vi "ctrlMain.vi"() -> ()   [LabVIEW 2012]
panel:
  out "Label":string
  in  "InitDevices":bool
  out "数值":i32
  out "remote address":string caption="远程地址"
  out "remote port":u16 caption="远程端口"
  out "data out":string
  in  "StopTCP":bool
  in  "StopLoop":bool
  out "status changed":string
  out "REDY_THL5":bool caption="THL5"
  out "REDY_THL3":bool caption="THL3"
  out "REDY_THL6":bool caption="THL6"
  out "REDY_THL4":bool caption="THL4"
  out "REDY_THL2":bool caption="THL2"
  out "REDY_THL1":bool caption="THL1"
  out "REDY_PIZ":bool caption="PIZ"
  out "REDY_NPR":bool caption="NPR"
  out "REDY_NPM":bool caption="NPM"
  in  "选项卡控件 2":T1(tab)
  out "sz":bool
  out "sy":bool
  out "sx":bool
  in  "pz":dbl
  in  "py":dbl
  in  "px":dbl
  out "pxd":dbl
  in  "Sample_speed":dbl(slide) scale=0.01..10.0
  in  "x-":bool
  in  "x+":bool
  in  "y+":bool
  in  "y-":bool
  in  "z-":bool
  in  "z+":bool
  out "pyd":dbl
  out "pzd":dbl
  out "sM2y":bool
  out "sM2x":bool
  out "sM1y":bool
  out "sM1x":bool
  in  "M2xp":dbl
  in  "M1yp":dbl
  in  "M1xp":dbl
  out "M1xpd":dbl
  in  "M_speed":i16(slide) scale=10.0..2000.0
  in  "M1x-":bool
  in  "M1x+":bool
  in  "M1y+":bool
  in  "M1y-":bool
  in  "M2x-":bool
  in  "M2x+":bool
  out "M1ypd":dbl
  out "M2xpd":dbl
  out "M2ypd":dbl
  in  "M2y+":bool
  in  "M2y-":bool
  in  "M2yp":dbl
  out "Obj2s":bool
  out "Obj1s":bool
  out "Obj2pd":dbl
  in  "Obj2-":bool
  in  "Obj2+":bool
  in  "Obj1+":bool
  in  "Obj1-":bool
  in  "Obj_speed":dbl(slide) scale=0.01..10.0
  out "Obj1pd":dbl
  in  "Obj1p":dbl
  in  "Obj2p":dbl
  in  "PIp":dbl
  in  "PI_step":dbl(slide) scale=0.01..10.0
  in  "PI+":bool
  in  "PI-":bool
  out "PIpd":dbl
  out "PIs":bool
  in  "Optp":dbl
  in  "Opt-":bool
  in  "Opt+":bool
  out "Optpd":dbl
  out "NPRpd":dbl
  in  "NPR+":bool
  in  "NPR-":bool
  in  "Opt_speed":dbl(slide) scale=0.01..10.0
  in  "NPRp":dbl
  out "NPRs":bool
  out "Opts":bool
  in  "NPR_step":dbl(slide) scale=0.01..10.0
  out "字符串":string
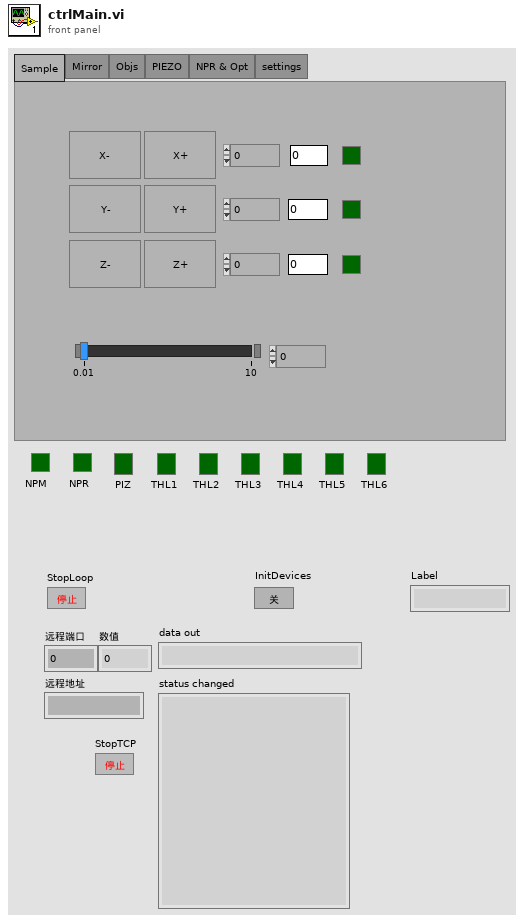
[diagram p1: front panel]
types:
  T1 = enum32{"Sample", "Mirror", "Objs", "PIEZO", "NPR & Opt", "settings"}
  T2 = enum16{"Standard", "Buffered", "CRLF", "Immediate"}
  T3 = cluster{"NPM_REDY":bool, "NPM_GETS1":bool, "NPM_GETP1":dbl, "NPM_GETV1":dbl, "NPR_REDY":bool, "NPR_GETS":bool, "NPR_GETP":dbl, "PIZ_REDY":bool, "PIZ_GETS":bool, "PIZ_GETP":dbl, "THL_REDY1":bool, "THL_REDY2":bool, "THL_REDY3":bool, "THL_REDY4":bool, "THL_REDY5":bool, "THL_REDY6":bool, "THL_GETS1":bool, "THL_GETS2":bool, "THL_GETS3":bool, "THL_GETS4":bool, "THL_GETS5":bool, "THL_GETS6":bool, "THL_GETP1":dbl, "THL_GETP2":dbl, "THL_GETP3":dbl, "THL_GETP4":dbl, "THL_GETP5":dbl, "THL_GETP6":dbl, "THL_GETV1":dbl, "THL_GETV2":dbl, "THL_GETV3":dbl, "THL_GETV4":dbl, "THL_GETV5":dbl, "THL_GETV6":dbl, "NPM_GETS2":bool, "NPM_GETS3":bool, "NPM_GETS4":bool, "NPM_GETP2":dbl, "NPM_GETP3":dbl, "NPM_GETP4":dbl, "NPM_GETV2":dbl, "NPM_GETV3":dbl, "NPM_GETV4":dbl}
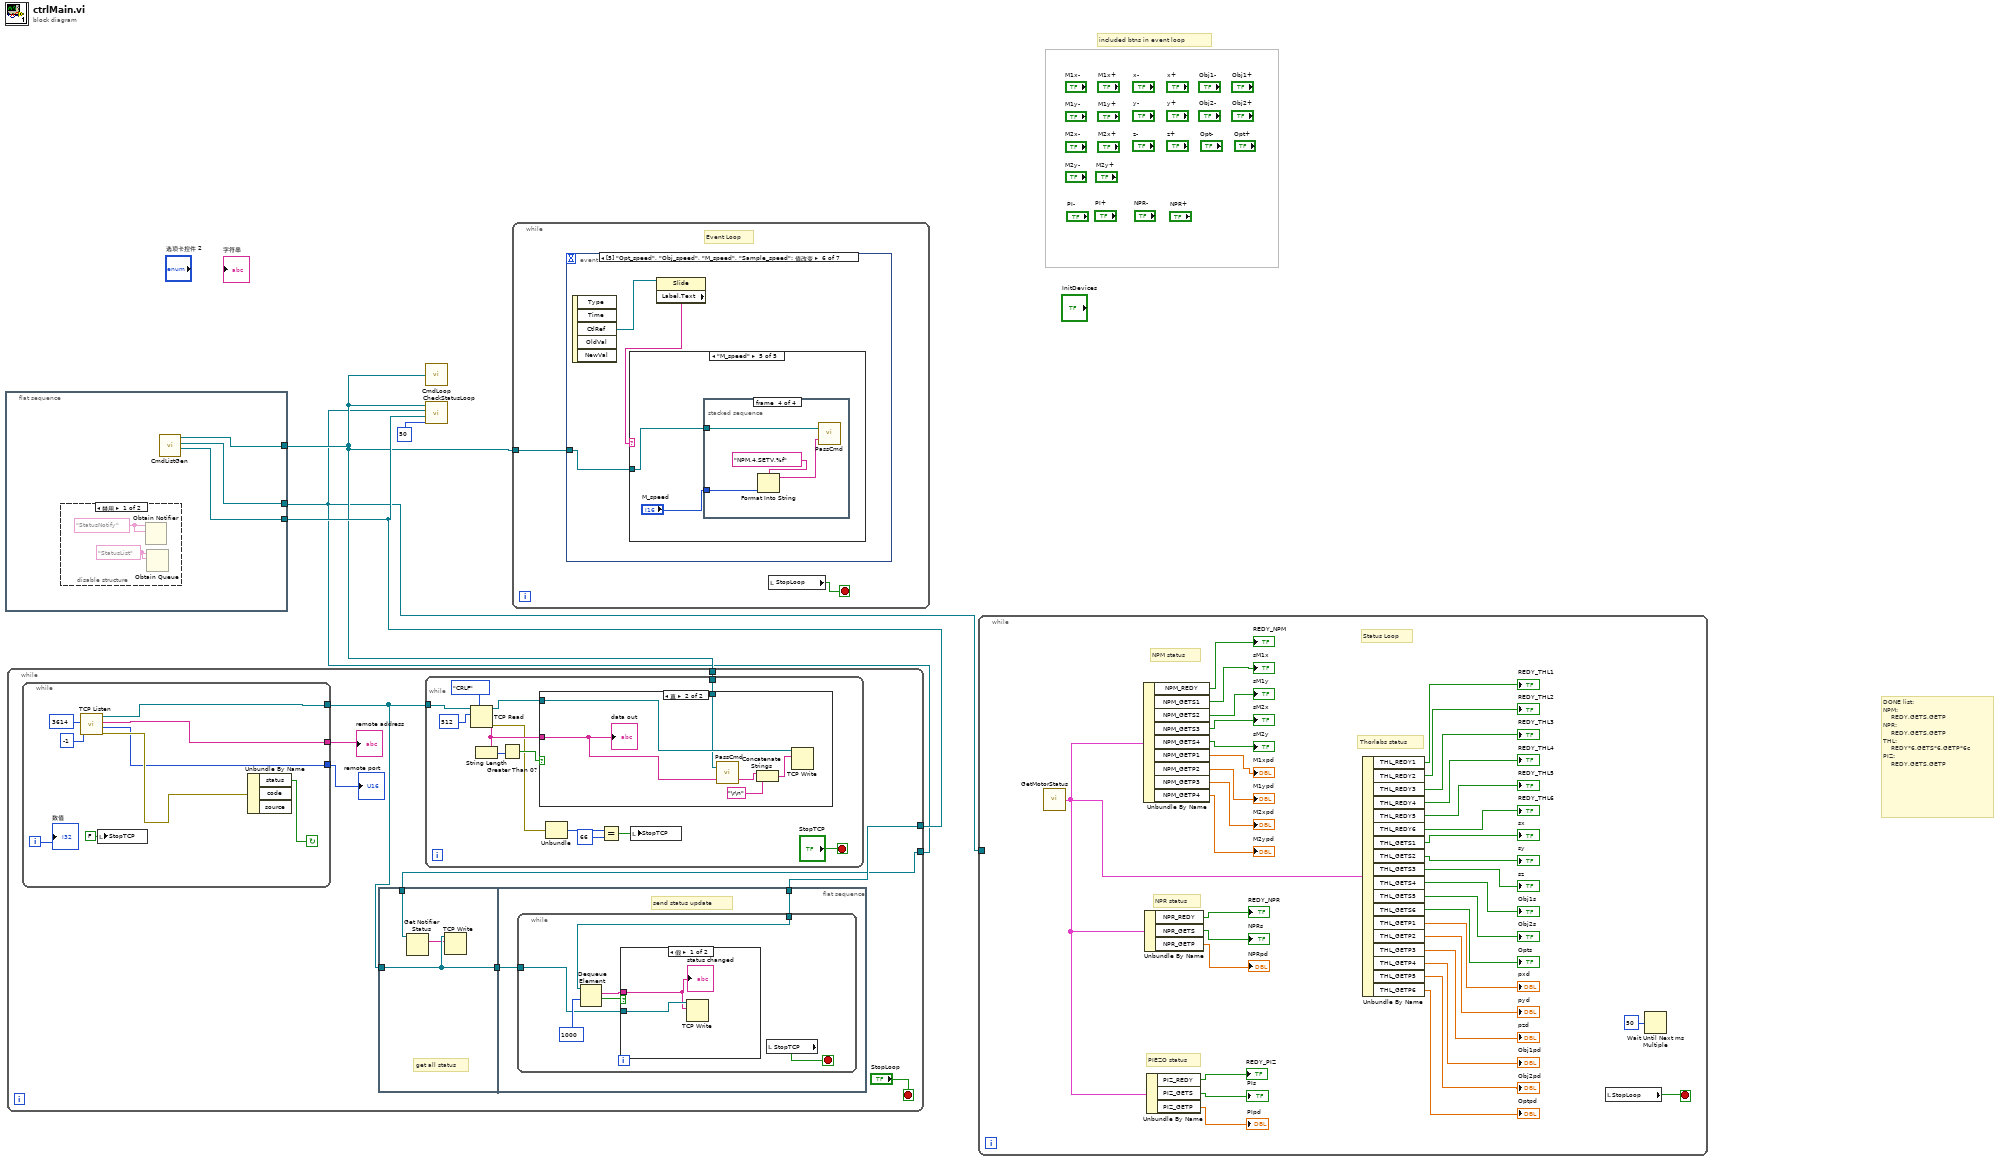
[diagram p0: block diagram]
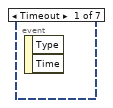
[diagram p2: hidden frame]
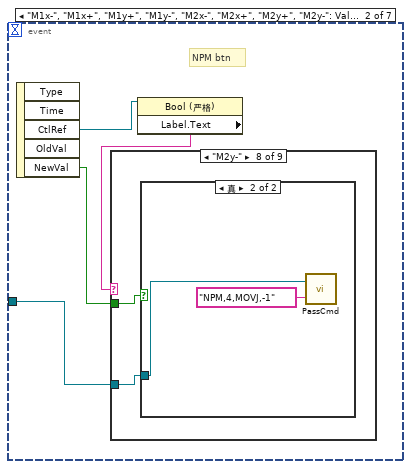
[diagram p3: hidden frame]
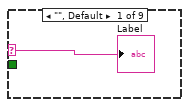
[diagram p4: hidden frame]
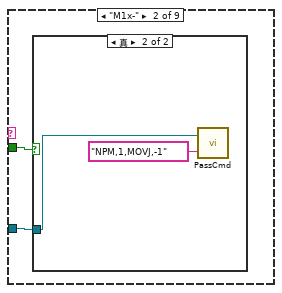
[diagram p5: hidden frame]
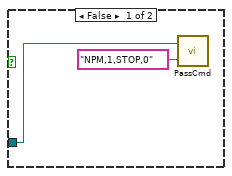
[diagram p6: hidden frame]
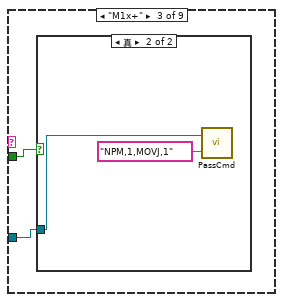
[diagram p7: hidden frame]
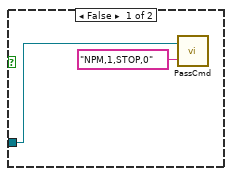
[diagram p8: hidden frame]
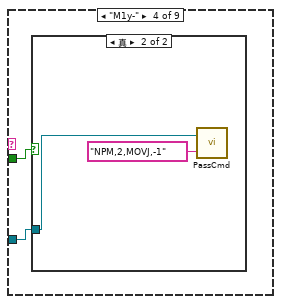
[diagram p9: hidden frame]
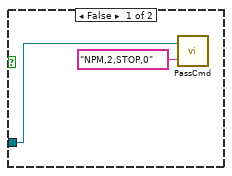
[diagram p10: hidden frame]
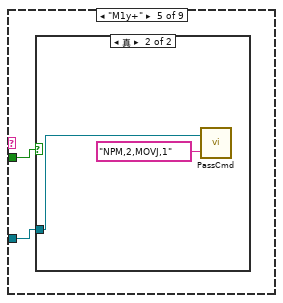
[diagram p11: hidden frame]
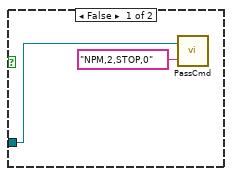
[diagram p12: hidden frame]
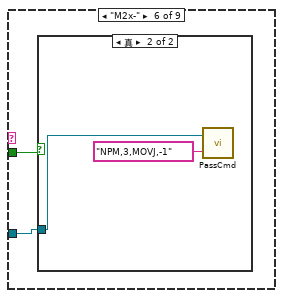
[diagram p13: hidden frame]
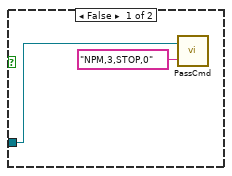
[diagram p14: hidden frame]
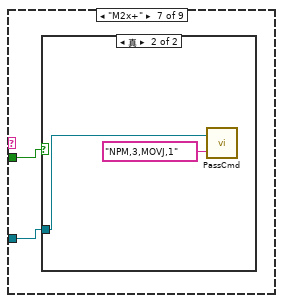
[diagram p15: hidden frame]
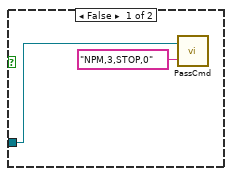
[diagram p16: hidden frame]
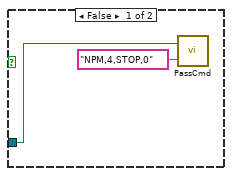
[diagram p17: hidden frame]
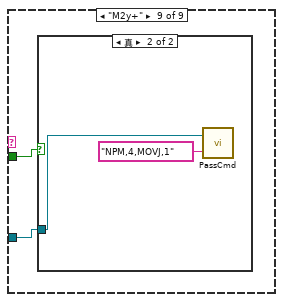
[diagram p18: hidden frame]
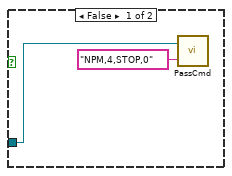
[diagram p19: hidden frame]
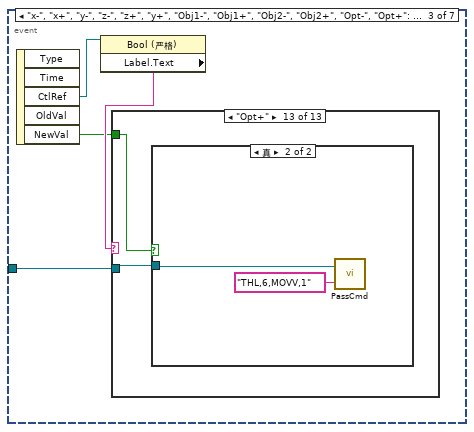
[diagram p20: hidden frame]
diagram:
  # "included btns in event loop"
  # "DONE list:\nNPM:\n    REDY,GETS,GETP\nNPR:\n    REDY,GETS,GETP\nTHL:\n    REDY*6,GETS*6,GETP*6c\nPIZ:\n    REDY,GETS,GETP"
  n1 = flat-sequence {
    tunnel: [w7] -> w2
    tunnel: [w5] -> w3
    tunnel: [w6] -> w1
    frame #0 {
      n2 = disable-structure shown="禁用" {
        frame Disabled {
          w8 = "StatusList" ("名称（未命名）")
          w9 = "StatusNotify" ("名称（未命名）")
          n3 = Obtain Notifier(name (unnamed)=w9, notification data type=w9) -> ()  [unwired: 2 in, 3 out]
          n4 = Obtain Queue(name (unnamed)=w8, element data type=w8) -> ()  [unwired: 3 in, 3 out]
        }
        frame Enabled {
        }
      }
      n5 = call "CmdListGen.vi"() -> ("MsgList"=w7:refnum<queue>, "StatusNotify"=w6:refnum<notifier>, "StatusList"=w5:refnum<queue>)  [unwired: 1 in, 1 out]
    }
  }
  n6 = while {
    tunnel: w2 -> [w15]
    tunnel: w3 -> [w12]
    tunnel: w1 -> [w10]
    stop <- "StopLoop" stop-if-true
    n7 = while {
      tunnel: [w56] -> w13
      tunnel: [w53] -> w17
      tunnel: [w52] -> w16
      i -> [w51]
      stop <- w54 continue-if-true
      n8 = call <vilib>:"TCP Listen.vi"("timeout ms (wait forever: -1)"=-1, "port"=u16 3614) -> ("error out"=w55:errorcluster, "remote port"=w52:u16, "remote address"=w53:string, "connection ID"=w56:refnum<k5>)  [unwired: 5 in, 1 out]
      n9 = local write "StopTCP"(FALSE ("停止 3")) -> ()
      n10 = Unbundle By Name(w55) -> ("status"=w54:bool)  [unwired: 2 out]
      "数值" <- w51
    }
    "remote address" <- w17
    "remote port" <- w16
    n11 = flat-sequence {
      tunnel: w13 -> [w19]
      tunnel: [w19] -> w11
      tunnel: w10 -> [w20]
      tunnel: w12 -> [w21]
      tunnel: w11 -> [w22]
      frame #0 {
        # "get all status"
        n12 = Get Notifier Status(notifier=w20) -> (current notification=w18:string)  [unwired: 1 in, 4 out]
        n13 = TCP Write(connection ID=w19, data in=w18) -> ()  [unwired: 2 in, 3 out]
      }
      frame #1 {
        # "send status update"
        n14 = while {
          tunnel: w22 -> [w24]
          tunnel: w21 -> [w28]
          stop <- w23 stop-if-true
          n15 = Dequeue Element(queue=w28, timeout in ms (-1)=1000 ("超时毫秒(-1)")) -> (element=w25:string, timed out?=w26:bool)  [unwired: 1 in, 2 out]
          n16 = case shown="假" w26 {
            tunnel: w25 -> [w29 _]
            tunnel: w24 -> [w30 _]
            frame False {
              n17 = TCP Write(connection ID=w30, data in=w29) -> ()  [unwired: 2 in, 3 out]
              "status changed" <- w29
            }
            frame True {
            }
          }
          n18 = local read "StopTCP"() -> (w23:bool)
        }
      }
    }
    n19 = while {
      tunnel: w13 -> [w35]
      tunnel: w15 -> [w33]
      stop <- "StopTCP" stop-if-true
      n20 = TCP Read(connection ID=w35, bytes to read=512 ("读取的字节"), 7:T2."CRLF" ("模式（标准）")) -> (connection ID out=w34:refnum<k5>, data out=w40:string, error out=w39:errorcluster)  [unwired: 2 in]
      n21 = String Length(string=w40) -> (length=w36:i32)
      n22 = Greater Than 0?(x=w36) -> (x > 0?=w41:bool)
      n23 = case shown="真" w41 {
        tunnel: w40 -> [_ w48]
        tunnel: w34 -> [_ w49]
        tunnel: w33 -> [_ w47]
        frame False {
        }
        frame True {
          n24 = call "PassCmd.vi"("cmd in"=w48, "list ref"=w47) -> ("str out"=w46:string)  [unwired: 1 out]
          n25 = Concatenate Strings(w46, "\r\n") -> (w45:string)
          n26 = TCP Write(connection ID=w49, data in=w45) -> ()  [unwired: 2 in, 3 out]
          "data out" <- w48
        }
      }
      n27 = Unbundle(w39) -> ("code"=w38:i32)  [unwired: 2 out]
      n28 = Equal?(x=w38, y=66) -> (x = y?=w31:bool)
      n29 = local write "StopTCP"(w31) -> ()
    }
  }
  n30 = call "CheckStatusLoop.vi"("loop time"=u32 50, "StatusListRef"=w3, "NotificationRef"=w1, "ListRef"=w2) -> ()  [unwired: 1 in]
  n31 = call "CmdLoop.vi"("ListRef"=w2) -> ()  [unwired: 1 out]
  n32 = while {
    tunnel: w2 -> [w59]
    stop <- w60 stop-if-true
    # "Event Loop"
    n33 = event shown="[5] \"Opt_speed\", \"Obj_speed\", \"M_speed\", \"Sample_speed\": 值改变" {
      selector: _ -> [_ _ _ _ _ _ _]
      dyn-events: _ -> [_ _ _ _ _ _ _]
      timeout: _ -> [_ _ _ _ _ _ _]
      tunnel: w59 -> [_ w63 w114 w192 w213 w264 w313]
      event Timeout {
        n34 = event-data() -> ()  [unwired: 1 in, 2 out]
      }
      event "M1x-", "M1x+", "M1y+", "M1y-", "M2x-", "M2x+", "M2y+", "M2y-": Value Change {
        # "NPM btn"
        n35 = event-data() -> ("CtlRef"=w62:refnum<vi>, "NewVal"=w64:bool)  [unwired: 1 in, 3 out]
        n36 = property class="Bool (严格)"(reference=w62) -> ("Label.Text"=w61:string)  [unwired: 1 in, 2 out]
        n37 = case shown="\"M2y-\"" w61 {
          selector: w61 -> [w65 _ _ _ _ _ _ _ _]
          tunnel: w64 -> [_ w67 w73 w79 w85 w91 w97 w103 w109]
          tunnel: w63 -> [_ w66 w72 w78 w84 w90 w96 w102 w108]
          frame "", Default {
            "Label" <- w65
          }
          frame "M1x-" {
            n38 = case shown="真" w67 {
              tunnel: w66 -> [w68 w70]
              frame False {
                n39 = call "PassCmd.vi"("cmd in"="NPM,1,STOP,0", "list ref"=w68) -> ()  [unwired: 2 out]
              }
              frame True {
                n40 = call "PassCmd.vi"("cmd in"="NPM,1,MOVJ,-1", "list ref"=w70) -> ()  [unwired: 2 out]
              }
            }
          }
          frame "M1x+" {
            n41 = case shown="真" w73 {
              tunnel: w72 -> [w74 w76]
              frame False {
                n42 = call "PassCmd.vi"("cmd in"="NPM,1,STOP,0", "list ref"=w74) -> ()  [unwired: 2 out]
              }
              frame True {
                n43 = call "PassCmd.vi"("cmd in"="NPM,1,MOVJ,1", "list ref"=w76) -> ()  [unwired: 2 out]
              }
            }
          }
          frame "M1y-" {
            n44 = case shown="真" w79 {
              tunnel: w78 -> [w80 w82]
              frame False {
                n45 = call "PassCmd.vi"("cmd in"="NPM,2,STOP,0", "list ref"=w80) -> ()  [unwired: 2 out]
              }
              frame True {
                n46 = call "PassCmd.vi"("cmd in"="NPM,2,MOVJ,-1", "list ref"=w82) -> ()  [unwired: 2 out]
              }
            }
          }
          frame "M1y+" {
            n47 = case shown="真" w85 {
              tunnel: w84 -> [w86 w88]
              frame False {
                n48 = call "PassCmd.vi"("cmd in"="NPM,2,STOP,0", "list ref"=w86) -> ()  [unwired: 2 out]
              }
              frame True {
                n49 = call "PassCmd.vi"("cmd in"="NPM,2,MOVJ,1", "list ref"=w88) -> ()  [unwired: 2 out]
              }
            }
          }
          frame "M2x-" {
            n50 = case shown="真" w91 {
              tunnel: w90 -> [w92 w94]
              frame False {
                n51 = call "PassCmd.vi"("cmd in"="NPM,3,STOP,0", "list ref"=w92) -> ()  [unwired: 2 out]
              }
              frame True {
                n52 = call "PassCmd.vi"("cmd in"="NPM,3,MOVJ,-1", "list ref"=w94) -> ()  [unwired: 2 out]
              }
            }
          }
          frame "M2x+" {
            n53 = case shown="真" w97 {
              tunnel: w96 -> [w98 w100]
              frame False {
                n54 = call "PassCmd.vi"("cmd in"="NPM,3,STOP,0", "list ref"=w98) -> ()  [unwired: 2 out]
              }
              frame True {
                n55 = call "PassCmd.vi"("cmd in"="NPM,3,MOVJ,1", "list ref"=w100) -> ()  [unwired: 2 out]
              }
            }
          }
          frame "M2y-" {
            n56 = case shown="真" w103 {
              tunnel: w102 -> [w104 w106]
              frame False {
                n57 = call "PassCmd.vi"("cmd in"="NPM,4,STOP,0", "list ref"=w104) -> ()  [unwired: 2 out]
              }
              frame True {
                n58 = call "PassCmd.vi"("cmd in"="NPM,4,MOVJ,-1", "list ref"=w106) -> ()  [unwired: 2 out]
              }
            }
          }
          frame "M2y+" {
            n59 = case shown="真" w109 {
              tunnel: w108 -> [w110 w112]
              frame False {
                n60 = call "PassCmd.vi"("cmd in"="NPM,4,STOP,0", "list ref"=w110) -> ()  [unwired: 2 out]
              }
              frame True {
                n61 = call "PassCmd.vi"("cmd in"="NPM,4,MOVJ,1", "list ref"=w112) -> ()  [unwired: 2 out]
              }
            }
          }
        }
      }
      event "x-", "x+", "y-", "z-", "z+", "y+", "Obj1-", "Obj1+", "Obj2-", "Obj2+", "Opt-", "Opt+": Value Change {
        n62 = event-data() -> ("CtlRef"=w117:refnum<vi>, "NewVal"=w115:bool)  [unwired: 1 in, 3 out]
        n63 = property class="Bool (严格)"(reference=w117) -> ("Label.Text"=w116:string)  [unwired: 1 in, 2 out]
        n64 = case shown="\"Opt+\"" w116 {
          tunnel: w115 -> [_ w119 w125 w131 w137 w143 w149 w155 w161 w167 w173 w179 w185]
          tunnel: w114 -> [_ w118 w124 w130 w136 w142 w148 w154 w160 w166 w172 w178 w184]
          frame "", Default {
          }
          frame "x-" {
            n65 = case shown="真" w119 {
              tunnel: w118 -> [w120 w122]
              frame False {
                n66 = call "PassCmd.vi"("cmd in"="THL,1,STOP,0", "list ref"=w120) -> ()  [unwired: 2 out]
              }
              frame True {
                n67 = call "PassCmd.vi"("cmd in"="THL,1,MOVV,-1", "list ref"=w122) -> ()  [unwired: 2 out]
              }
            }
          }
          frame "x+" {
            n68 = case shown="真" w125 {
              tunnel: w124 -> [w126 w128]
              frame False {
                n69 = call "PassCmd.vi"("cmd in"="THL,1,STOP,0", "list ref"=w126) -> ()  [unwired: 2 out]
              }
              frame True {
                n70 = call "PassCmd.vi"("cmd in"="THL,1,MOVV,1", "list ref"=w128) -> ()  [unwired: 2 out]
              }
            }
          }
          frame "y-" {
            n71 = case shown="真" w131 {
              tunnel: w130 -> [w132 w134]
              frame False {
                n72 = call "PassCmd.vi"("cmd in"="THL,2,STOP,0", "list ref"=w132) -> ()  [unwired: 2 out]
              }
              frame True {
                n73 = call "PassCmd.vi"("cmd in"="THL,2,MOVV,-1", "list ref"=w134) -> ()  [unwired: 2 out]
              }
            }
          }
          frame "y+" {
            n74 = case shown="真" w137 {
              tunnel: w136 -> [w138 w140]
              frame False {
                n75 = call "PassCmd.vi"("cmd in"="THL,2,STOP,0", "list ref"=w138) -> ()  [unwired: 2 out]
              }
              frame True {
                n76 = call "PassCmd.vi"("cmd in"="THL,2,MOVV,1", "list ref"=w140) -> ()  [unwired: 2 out]
              }
            }
          }
          frame "z-" {
            n77 = case shown="真" w143 {
              tunnel: w142 -> [w144 w146]
              frame False {
                n78 = call "PassCmd.vi"("cmd in"="THL,3,STOP,0", "list ref"=w144) -> ()  [unwired: 2 out]
              }
              frame True {
                n79 = call "PassCmd.vi"("cmd in"="THL,3,MOVV,-1", "list ref"=w146) -> ()  [unwired: 2 out]
              }
            }
          }
          frame "z+" {
            n80 = case shown="真" w149 {
              tunnel: w148 -> [w150 w152]
              frame False {
                n81 = call "PassCmd.vi"("cmd in"="THL,3,STOP,0", "list ref"=w150) -> ()  [unwired: 2 out]
              }
              frame True {
                n82 = call "PassCmd.vi"("cmd in"="THL,3,MOVV,1", "list ref"=w152) -> ()  [unwired: 2 out]
              }
            }
          }
          frame "Obj1-" {
            n83 = case shown="真" w155 {
              tunnel: w154 -> [w156 w158]
              frame False {
                n84 = call "PassCmd.vi"("cmd in"="THL,4,STOP,0", "list ref"=w156) -> ()  [unwired: 2 out]
              }
              frame True {
                n85 = call "PassCmd.vi"("cmd in"="THL,4,MOVV,-1", "list ref"=w158) -> ()  [unwired: 2 out]
              }
            }
          }
          frame "Obj1+" {
            n86 = case shown="真" w161 {
              tunnel: w160 -> [w162 w164]
              frame False {
                n87 = call "PassCmd.vi"("cmd in"="THL,4,STOP,0", "list ref"=w162) -> ()  [unwired: 2 out]
              }
              frame True {
                n88 = call "PassCmd.vi"("cmd in"="THL,4,MOVV,1", "list ref"=w164) -> ()  [unwired: 2 out]
              }
            }
          }
          frame "Obj2-" {
            n89 = case shown="真" w167 {
              tunnel: w166 -> [w168 w170]
              frame False {
                n90 = call "PassCmd.vi"("cmd in"="THL,5,STOP,0", "list ref"=w168) -> ()  [unwired: 2 out]
              }
              frame True {
                n91 = call "PassCmd.vi"("cmd in"="THL,5,MOVV,-1", "list ref"=w170) -> ()  [unwired: 2 out]
              }
            }
          }
          frame "Obj2+" {
            n92 = case shown="真" w173 {
              tunnel: w172 -> [w174 w176]
              frame False {
                n93 = call "PassCmd.vi"("cmd in"="THL,5,STOP,0", "list ref"=w174) -> ()  [unwired: 2 out]
              }
              frame True {
                n94 = call "PassCmd.vi"("cmd in"="THL,5,MOVV,1", "list ref"=w176) -> ()  [unwired: 2 out]
              }
            }
          }
          frame "Opt-" {
            n95 = case shown="假" w179 {
              tunnel: w178 -> [w180 w182]
              frame False {
                n96 = call "PassCmd.vi"("cmd in"="THL,6,STOP,0", "list ref"=w180) -> ()  [unwired: 2 out]
              }
              frame True {
                n97 = call "PassCmd.vi"("cmd in"="THL,6,MOVV,-1", "list ref"=w182) -> ()  [unwired: 2 out]
              }
            }
          }
          frame "Opt+" {
            n98 = case shown="真" w185 {
              tunnel: w184 -> [w186 w188]
              frame False {
                n99 = call "PassCmd.vi"("cmd in"="THL,6,STOP,0", "list ref"=w186) -> ()  [unwired: 2 out]
              }
              frame True {
                n100 = call "PassCmd.vi"("cmd in"="THL,6,MOVV,1", "list ref"=w188) -> ()  [unwired: 2 out]
              }
            }
          }
        }
      }
      event "PI+", "PI-", "NPR+", "NPR-": Mouse Up {
        n101 = event-data() -> ("CtlRef"=w194:refnum<vi>)  [unwired: 1 in, 6 out]
        n102 = property class="Bool (严格)"(reference=w194) -> ("Label.Text"=w193:string)  [unwired: 1 in, 2 out]
        n103 = case shown="\"PI+\"" w193 {
          tunnel: w192 -> [_ w198 w201 w205 w210]
          tunnel: "PI_step" -> [_ w196 w200 _ _]
          tunnel: "NPR_step" -> [_ _ _ w204 w208]
          frame "假", Default {
          }
          frame "PI+" {
            n104 = Format Into String(format string="PIZ,1,MOVR,%f" ("格式字符串"), w196) -> (resulting string=w195:string)  [unwired: 2 in, 1 out]
            n105 = call "PassCmd.vi"("cmd in"=w195, "list ref"=w198) -> ()  [unwired: 2 out]
          }
          frame "PI-" {
            n106 = Negate(x=w200) -> (-x=w199:dbl)
            n107 = Format Into String(format string="PIZ,1,MOVR,%f" ("格式字符串"), w199) -> (resulting string=w203:string)  [unwired: 2 in, 1 out]
            n108 = call "PassCmd.vi"("cmd in"=w203, "list ref"=w201) -> ()  [unwired: 2 out]
          }
          frame "NPR+" {
            n109 = Format Into String(format string="NPR,1,MOVR,%f" ("格式字符串"), w204) -> (resulting string=w207:string)  [unwired: 2 in, 1 out]
            n110 = call "PassCmd.vi"("cmd in"=w207, "list ref"=w205) -> ()  [unwired: 2 out]
          }
          frame "NPR-" {
            n111 = Negate(x=w208) -> (-x=w209:dbl)
            n112 = Format Into String(format string="NPR,1,MOVR,%f" ("格式字符串"), w209) -> (resulting string=w212:string)  [unwired: 2 in, 1 out]
            n113 = call "PassCmd.vi"("cmd in"=w212, "list ref"=w210) -> ()  [unwired: 2 out]
          }
        }
      }
      event "px", "py", "pz", "Obj1p", "Obj2p", "Optp", "M1xp", "M1yp", "M2xp", "M2yp", "PIp", "NPRp": Value Change {
        n114 = event-data() -> ("CtlRef"=w215:refnum<vi>)  [unwired: 1 in, 4 out]
        n115 = property class="DigNum (严格)"(reference=w215) -> ("Label.Text"=w214:string)  [unwired: 1 in, 2 out]
        n116 = case shown="\"PIp\"" w214 {
          tunnel: w213 -> [_ w217 w221 w225 w229 w233 w237 w240 w245 w249 w252 w257 w261]
          frame "假", Default {
          }
          frame "px" {
            n117 = Format Into String(format string="THL,1,MOVP,%f" ("格式字符串"), "px") -> (resulting string=w218:string)  [unwired: 2 in, 1 out]
            n118 = call "PassCmd.vi"("cmd in"=w218, "list ref"=w217) -> ()  [unwired: 2 out]
          }
          frame "py" {
            n119 = Format Into String(format string="THL,2,MOVP,%f" ("格式字符串"), "py") -> (resulting string=w222:string)  [unwired: 2 in, 1 out]
            n120 = call "PassCmd.vi"("cmd in"=w222, "list ref"=w221) -> ()  [unwired: 2 out]
          }
          frame "pz" {
            n121 = Format Into String(format string="THL,3,MOVP,%f" ("格式字符串"), "pz") -> (resulting string=w227:string)  [unwired: 2 in, 1 out]
            n122 = call "PassCmd.vi"("cmd in"=w227, "list ref"=w225) -> ()  [unwired: 2 out]
          }
          frame "Obj1p" {
            n123 = Format Into String(format string="THL,4,MOVP,%f" ("格式字符串"), "Obj1p") -> (resulting string=w230:string)  [unwired: 2 in, 1 out]
            n124 = call "PassCmd.vi"("cmd in"=w230, "list ref"=w229) -> ()  [unwired: 2 out]
          }
          frame "Obj2p" {
            n125 = Format Into String(format string="THL,5,MOVP,%f" ("格式字符串"), "Obj2p") -> (resulting string=w235:string)  [unwired: 2 in, 1 out]
            n126 = call "PassCmd.vi"("cmd in"=w235, "list ref"=w233) -> ()  [unwired: 2 out]
          }
          frame "Optp" {
            n127 = Format Into String(format string="THL,6,MOVP,%f" ("格式字符串"), "Optp") -> (resulting string=w238:string)  [unwired: 2 in, 1 out]
            n128 = call "PassCmd.vi"("cmd in"=w238, "list ref"=w237) -> ()  [unwired: 2 out]
          }
          frame "M1xp" {
            n129 = Format Into String(format string="NPM,1,MOVP,%f" ("格式字符串"), "M1xp") -> (resulting string=w243:string)  [unwired: 2 in, 1 out]
            n130 = call "PassCmd.vi"("cmd in"=w243, "list ref"=w240) -> ()  [unwired: 2 out]
          }
          frame "M1yp" {
            n131 = Format Into String(format string="NPM,2,MOVP,%f" ("格式字符串"), "M1yp") -> (resulting string=w246:string)  [unwired: 2 in, 1 out]
            n132 = call "PassCmd.vi"("cmd in"=w246, "list ref"=w245) -> ()  [unwired: 2 out]
          }
          frame "M2xp" {
            n133 = Format Into String(format string="NPM,3,MOVP,%f" ("格式字符串"), "M2xp") -> (resulting string=w251:string)  [unwired: 2 in, 1 out]
            n134 = call "PassCmd.vi"("cmd in"=w251, "list ref"=w249) -> ()  [unwired: 2 out]
          }
          frame "M2yp" {
            n135 = Format Into String(format string="NPM,4,MOVP,%f" ("格式字符串"), "M2yp") -> (resulting string=w254:string)  [unwired: 2 in, 1 out]
            n136 = call "PassCmd.vi"("cmd in"=w254, "list ref"=w252) -> ()  [unwired: 2 out]
          }
          frame "PIp" {
            n137 = Format Into String(format string="PIZ,1,MOVP,%f" ("格式字符串"), "PIp") -> (resulting string=w259:string)  [unwired: 2 in, 1 out]
            n138 = call "PassCmd.vi"("cmd in"=w259, "list ref"=w257) -> ()  [unwired: 2 out]
          }
          frame "NPRp" {
            n139 = Format Into String(format string="NPR,1,MOVP,%f" ("格式字符串"), "NPRp") -> (resulting string=w262:string)  [unwired: 2 in, 1 out]
            n140 = call "PassCmd.vi"("cmd in"=w262, "list ref"=w261) -> ()  [unwired: 2 out]
          }
        }
      }
      event "Opt_speed", "Obj_speed", "M_speed", "Sample_speed": Value Change {
        n141 = event-data() -> ("CtlRef"=w266:refnum<vi>)  [unwired: 1 in, 4 out]
        n142 = property class="Slide"(reference=w266) -> ("Label.Text"=w265:string)  [unwired: 1 in, 2 out]
        n143 = case shown="\"M_speed\"" w265 {
          tunnel: w264 -> [_ w268 w282 w292 w296]
          frame "假", Default {
          }
          frame "Sample_speed" {
            n144 = stacked-sequence {
              tunnel: w268 -> [w270 w274 w278]
              tunnel: "Sample_speed" -> [w269 w273 w277]
              frame #0 {
                n145 = Format Into String(format string="THL,1,SETV,%f" ("格式字符串"), w269) -> (resulting string=w272:string)  [unwired: 2 in, 1 out]
                n146 = call "PassCmd.vi"("cmd in"=w272, "list ref"=w270) -> ()  [unwired: 2 out]
              }
              frame #1 {
                n147 = Format Into String(format string="THL,2,SETV,%f" ("格式字符串"), w273) -> (resulting string=w276:string)  [unwired: 2 in, 1 out]
                n148 = call "PassCmd.vi"("cmd in"=w276, "list ref"=w274) -> ()  [unwired: 2 out]
              }
              frame #2 {
                n149 = Format Into String(format string="THL,3,SETV,%f" ("格式字符串"), w277) -> (resulting string=w280:string)  [unwired: 2 in, 1 out]
                n150 = call "PassCmd.vi"("cmd in"=w280, "list ref"=w278) -> ()  [unwired: 2 out]
              }
            }
          }
          frame "Obj_speed" {
            n151 = stacked-sequence {
              tunnel: w282 -> [w284 w288]
              tunnel: "Obj_speed" -> [w283 w287]
              frame #0 {
                n152 = Format Into String(format string="THL,4,SETV,%f" ("格式字符串"), w283) -> (resulting string=w286:string)  [unwired: 2 in, 1 out]
                n153 = call "PassCmd.vi"("cmd in"=w286, "list ref"=w284) -> ()  [unwired: 2 out]
              }
              frame #1 {
                n154 = Format Into String(format string="THL,5,SETV,%f" ("格式字符串"), w287) -> (resulting string=w290:string)  [unwired: 2 in, 1 out]
                n155 = call "PassCmd.vi"("cmd in"=w290, "list ref"=w288) -> ()  [unwired: 2 out]
              }
            }
          }
          frame "Opt_speed" {
            n156 = Format Into String(format string="THL,6,SETV,%f" ("格式字符串"), "Opt_speed") -> (resulting string=w293:string)  [unwired: 2 in, 1 out]
            n157 = call "PassCmd.vi"("cmd in"=w293, "list ref"=w292) -> ()  [unwired: 2 out]
          }
          frame "M_speed" {
            n158 = stacked-sequence {
              tunnel: w296 -> [w298 w302 w306 w310]
              tunnel: "M_speed" -> [w297 w301 w305 w309]
              frame #0 {
                n159 = Format Into String(format string="NPM,1,SETV,%f" ("格式字符串"), w297) -> (resulting string=w299:string)  [unwired: 2 in, 1 out]
                n160 = call "PassCmd.vi"("cmd in"=w299, "list ref"=w298) -> ()  [unwired: 2 out]
              }
              frame #1 {
                n161 = Format Into String(format string="NPM,2,SETV,%f" ("格式字符串"), w301) -> (resulting string=w303:string)  [unwired: 2 in, 1 out]
                n162 = call "PassCmd.vi"("cmd in"=w303, "list ref"=w302) -> ()  [unwired: 2 out]
              }
              frame #2 {
                n163 = Format Into String(format string="NPM,3,SETV,%f" ("格式字符串"), w305) -> (resulting string=w307:string)  [unwired: 2 in, 1 out]
                n164 = call "PassCmd.vi"("cmd in"=w307, "list ref"=w306) -> ()  [unwired: 2 out]
              }
              frame #3 {
                n165 = Format Into String(format string="NPM,4,SETV,%f" ("格式字符串"), w309) -> (resulting string=w311:string)  [unwired: 2 in, 1 out]
                n166 = call "PassCmd.vi"("cmd in"=w311, "list ref"=w310) -> ()  [unwired: 2 out]
              }
            }
          }
        }
      }
      event "InitDevices": Mouse Up {
        n167 = event-data() -> ()  [unwired: 1 in, 7 out]
        n168 = call "PassCmd.vi"("cmd in"="NPM,1,INIT,0", "list ref"=w313) -> ()  [unwired: 2 out]
      }
    }
    n169 = local read "StopLoop"() -> (w60:bool)
  }
  n170 = while {
    tunnel: w1 -> [_]
    stop <- w350 stop-if-true
    # "Thorlabs status"
    # "PIEZO status"
    # "NPR status"
    # "NPM status"
    # "Status Loop"
    n171 = call "GetMotorStatus.vi"() -> ("status"=w333:T3)  [unwired: 1 in]
    n172 = Unbundle By Name(w333) -> ("NPM_REDY"=→"REDY_NPM":bool, "NPM_GETS1"=→"sM1x":bool, "NPM_GETS2"=→"sM1y":bool, "NPM_GETS3"=→"sM2x":bool, "NPM_GETS4"=→"sM2y":bool, "NPM_GETP1"=→"M1xpd":dbl, "NPM_GETP2"=→"M1ypd":dbl, "NPM_GETP3"=→"M2xpd":dbl, "NPM_GETP4"=→"M2ypd":dbl)
    n173 = Unbundle By Name(w333) -> ("NPR_REDY"=→"REDY_NPR":bool, "NPR_GETS"=→"NPRs":bool, "NPR_GETP"=→"NPRpd":dbl)
    n174 = Unbundle By Name(w333) -> ("PIZ_REDY"=→"REDY_PIZ":bool, "PIZ_GETS"=→"PIs":bool, "PIZ_GETP"=→"PIpd":dbl)
    n175 = Unbundle By Name(w333) -> ("THL_REDY1"=→"REDY_THL1":bool, "THL_REDY2"=→"REDY_THL2":bool, "THL_REDY3"=→"REDY_THL3":bool, "THL_REDY4"=→"REDY_THL4":bool, "THL_REDY5"=→"REDY_THL5":bool, "THL_REDY6"=→"REDY_THL6":bool, "THL_GETS1"=→"sx":bool, "THL_GETS2"=→"sy":bool, "THL_GETS3"=→"sz":bool, "THL_GETS4"=→"Obj1s":bool, "THL_GETS5"=→"Obj2s":bool, "THL_GETS6"=→"Opts":bool, "THL_GETP1"=→"pxd":dbl, "THL_GETP2"=→"pyd":dbl, "THL_GETP3"=→"pzd":dbl, "THL_GETP4"=→"Obj1pd":dbl, "THL_GETP5"=→"Obj2pd":dbl, "THL_GETP6"=→"Optpd":dbl)
    n176 = local read "StopLoop"() -> (w350:bool)
    n177 = Wait Until Next ms Multiple(millisecond multiple=u32 50 ("毫秒倍数")) -> ()  [unwired: 1 out]
  }
